vi "Get Class Name.vi"(11 "lvclass":refnum<class>) -> (3 "Class Name":string)   [LabVIEW 2014]
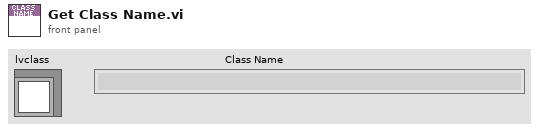
[diagram p1: front panel]
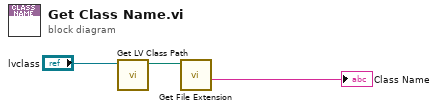
[diagram p0: block diagram]
diagram:
  n1 = call <vilib>:"Get LV Class Path.vi"("object"="lvclass") -> ("class path"=w2:path)  [unwired: 9 in, 1 out]
  n2 = call <vilib>:"Get File Extension.vi"("file"=w2) -> ("filename without extension"=→"Class Name":string)  [unwired: 7 in, 3 out]
